vi "MRC Init String With Length.vi"(8 "error in (no error)":errorcluster, 9 "length":i64, 10 "utf8String":string, 11 "mrcString":cluster{"str":u64, "len":i64}) -> (0 "error out":errorcluster, 2 "str":string, 3 "mrcString out":cluster{"str":u64, "len":i64})   [LabVIEW 2026, in "MrcLib.lvlib"]
doc: "void MRC_CALLCONV MRC_InitStringWithLength(struct MRC_String* mrcString,\n const char* utf8String, size_t length);"
uses:
  MrcLib.lvlib
  MrcLib.dll
  <vilib>/Utility/importsl/GetValueByPointer/GetValueByPointer.xnode
  <vilib>/Utility/importsl/GetValueByPointer/datatype.ctl
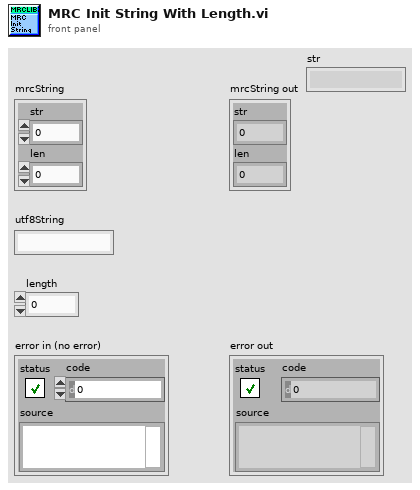
[diagram p1: front panel]
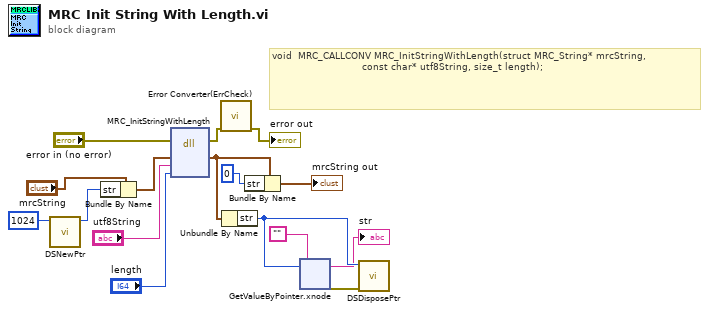
[diagram p0: block diagram]
diagram:
  # "void  MRC_CALLCONV MRC_InitStringWithLength(struct MRC_String* mrcString,\n                              const char* utf8String, size_t length);"
  n1 = call <vilib>:"DSNewPtr.vi"("Size"=u64 1024) -> ("Pointer"=w14:u64)  [unwired: 9 in, 1 out]
  n2 = Bundle By Name(cluster="mrcString", "str"=w14) -> (w13:cluster{"str":u64, "len":i64})
  n3 = dll-call lib="MrcLib.*" fn="MRC_InitStringWithLength"(error in="error in (no error)", "mrcString"=w13, "utf8String"="utf8String", "length"="length") -> (error out=w2:errorcluster, "mrcString"=w8:cluster{"str":u64, "len":i64})  [unwired: 5 in, 1 out]
  n4 = call <vilib>:"Error Converter(ErrCheck).vi"("error in (no error)"=w2) -> ("error out"=→"error out":errorcluster)  [unwired: 10 in]
  n5 = Unbundle By Name(w8) -> ("str"=w11:u64)
  n6 = Bundle By Name(cluster=w8, "str"=u64 0) -> (→"mrcString out":cluster{"str":u64, "len":i64})
  n7 = xnode "GetValueByPointer.xnode"("Pointer"=w11, "InputType"="") -> ("Output"=→"str":string, "ErrorOut"=w12:errorcluster)  [unwired: 2 in]
  n8 = call <vilib>:"DSDisposePtr.vi"("error in (no error)"=w12, "Pointer"=w11) -> ()  [unwired: 9 in, 1 out]
